vi "Value.vi"(8 "error in (no error)":errorcluster, 11 "ColumnPanel in":refnum<class "ColumnPanel.lvclass">) -> (0 "error out":errorcluster, 2 "Field Config":T1)   [LabVIEW 2020, in "Conditum-Tools.lvlib" / "ColumnPanel.lvclass"]
uses:
  ColumnPanel.lvclass
  Field Config.ctl
  Conditum-Clone/Columns/Type/Type.lvclass
  Accessors.ctl
  Accessor Scope.ctl
  Field Event Data.ctl
  ColumnPanel.lvclass/ColumnPanel.ctl
  Conditum-Tools.lvlib
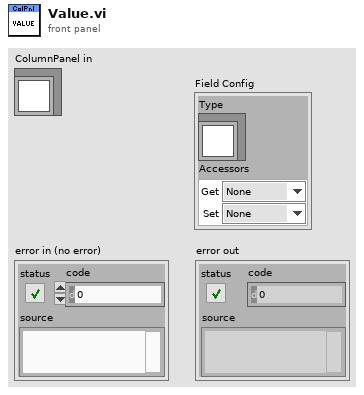
[diagram p1: front panel]
types:
  T1 = typedef "Conditum-Tools.lvlib/Field Config.ctl" = cluster{"Type":refnum<class "Type.lvclass">, "Accessors":T2}
  T2 = typedef "Conditum-Tools.lvlib/Accessors.ctl" = cluster{"Get":T3, "Set":T3}
  T3 = typedef "Conditum-Tools.lvlib/Accessor Scope.ctl" = enum16{"None", "Public", "Protected", "Private"}
  T4 = typedef "Conditum-Tools.lvlib/ColumnPanel.lvclass/Field Event Data.ctl" = cluster{"Field Config":T1}
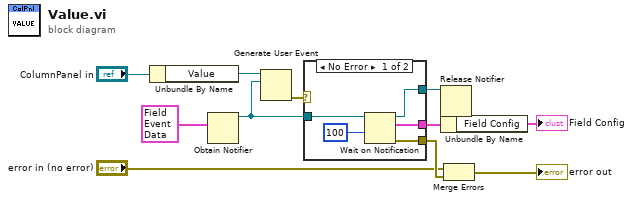
[diagram p0: block diagram]
diagram:
  n1 = Unbundle By Name("ColumnPanel in") -> ("Value"=w10:refnum<user-event>)
  n2 = Obtain Notifier(notification data type=T4 {"Field Config"={"Type"=refnum, "Accessors"={"Get"=enum."None", "Set"=enum."None"}}} ("Field Event Data")) -> (notifier out=w4:refnum<notifier>)  [unwired: 3 in, 2 out]
  n3 = Generate User Event(user event=w10, event data cluster=w4) -> (error out=w9:errorcluster)  [unwired: 2 in, 1 out]
  n4 = case shown="No Error" w9 {
    selector: w9 -> [_ w17]
    tunnel: w4 -> [w16 w18]
    tunnel: [w14 _] -> w2
    tunnel: [w13 w18] -> w8
    tunnel: [w12 w17] -> w7
    frame No Error {
      n5 = Wait on Notification(notifier=w16, timeout in ms (-1)=100) -> (notifier out=w13:refnum<notifier>, notification=w14:T4, error out=w12:errorcluster)  [unwired: 2 in, 1 out]
    }
    frame Error {
    }
  }
  n6 = Release Notifier(notifier=w8) -> ()  [unwired: 2 in, 3 out]
  n7 = Unbundle By Name(w2) -> ("Field Config"=→"Field Config":T1)
  n8 = Merge Errors("error in (no error)", w7) -> (→"error out":errorcluster)
